vi "Get Source Configuration List Size.vi"(8 "error in (no error)":errorcluster, 10 "Configuration List Name":string, 11 "VISA resource name":refnum<visa-resource-name>) -> (0 "error out":errorcluster, 2 "Source Configuration List Size":i32, 3 "VISA resource name out":refnum<visa-resource-name>)   [LabVIEW 2020, in "Keithley 2450.lvlib"]
doc: "Returns the size (number of configuration points) of a source configuration list"
uses:
  Keithley 2450.lvlib
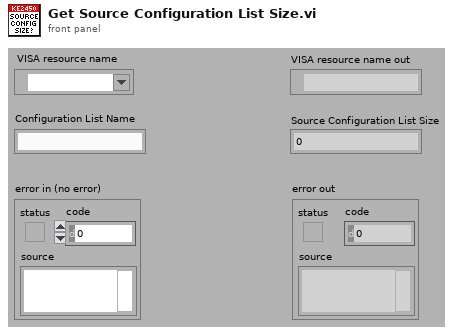
[diagram p1: front panel]
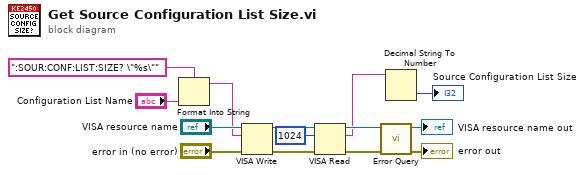
[diagram p0: block diagram]
diagram:
  n1 = Format Into String(format string=":SOUR:CONF:LIST:SIZE? \"%s\"", "Configuration List Name") -> (resulting string=w1:string)  [unwired: 2 in, 1 out]
  n2 = VISA Write(VISA resource name="VISA resource name", write buffer=w1, error in (no error)="error in (no error)") -> (VISA resource name out=w13:refnum<visa-resource-name>, error out=w14:errorcluster)  [unwired: 1 out]
  n3 = VISA Read(VISA resource name=w13, byte count=u32 1024, error in (no error)=w14) -> (VISA resource name out=w7:refnum<visa-resource-name>, read buffer=w2:string, error out=w6:errorcluster)  [unwired: 1 out]
  n4 = call "Error Query.vi"("error in (no error)"=w6, "VISA resource name"=w7) -> ("error out"=→"error out":errorcluster, "VISA resource name out"=→"VISA resource name out":refnum<visa-resource-name>)  [unwired: 8 out]
  n5 = Decimal String To Number(string=w2) -> (number=→"Source Configuration List Size":i32)  [unwired: 2 in, 1 out]
